vi "zadanie7_1.vi"() -> ()   [LabVIEW 2012]
panel:
  in  "Next":bool
  out "kolumna numer:":i32
  in  "Wpisz dane które mają pojawić się w kolumnie nr":string
  out "Dane na temat wykonawcy":T1 caption="Cluster"
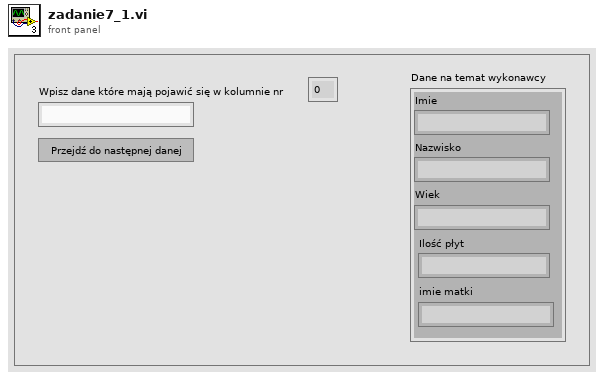
[diagram p1: front panel]
types:
  T1 = cluster{"Imie":string, "Nazwisko":string, "Wiek":string, "Ilość płyt":string, "imie matki":string}
  T2 = cluster{"[0]":string, "[1]":string, "[2]":string, "[3]":string, "[4]":string}
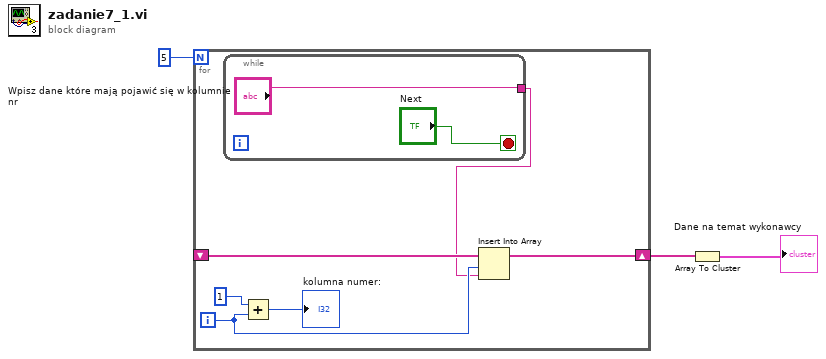
[diagram p0: block diagram]
diagram:
  n1 = for {
    N: 5 -> [_]
    shift-right: [w7] -> w2
    shift-left: _ -> [w6]
    i -> [w5]
    n2 = while {
      tunnel: ["Wpisz dane które mają pojawić się w kolumnie nr"] -> w4
      stop <- "Next" stop-if-true
    }
    n3 = Add(x=1, y=w5) -> (x+y=→"kolumna numer:":i32)
    n4 = Insert Into Array(array=w6, index=w5, new element=w4) -> (w7:string[])
  }
  n5 = Array To Cluster(array=w2) -> (cluster=→"Dane na temat wykonawcy":T2)
